vi "Raw_data.vi"(6 "y axis":dbl[](array[numeric]), 9 "dt/df":dbl, 10 "operation (0:open)":T1(ring), 11 "Data path":path) -> (2 "x axis":dbl[](array[numeric]), 3 "y data":dbl[](array[numeric]))   [LabVIEW 2021]
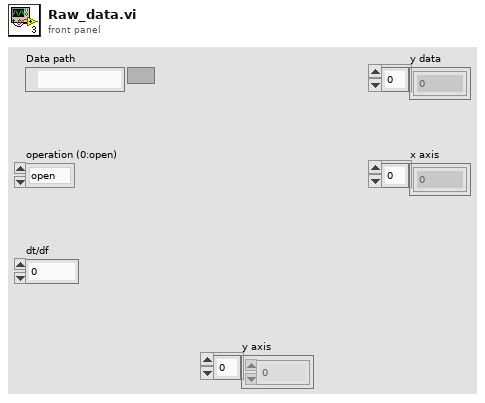
[diagram p1: front panel]
types:
  T1 = enum16{"open", "replace", "create", "open or create", "replace or create", "replace or create with confirmation"}
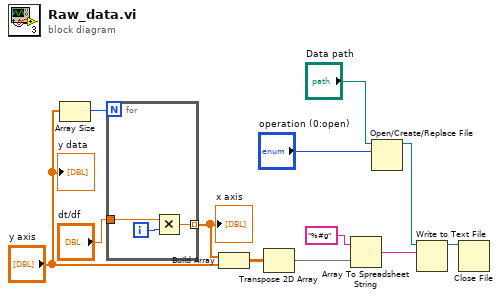
[diagram p0: block diagram]
diagram:
  n1 = Array Size(array="y axis") -> (size(s)=w7:i32)
  n2 = for {
    N: w7 -> [_]
    tunnel: [w15] -> w2 mode=indexing
    tunnel: "dt/df" -> [w13]
    i -> [w14]
    n3 = Multiply(x=w13, y=w14) -> (x*y=w15:dbl)
  }
  "x axis" <- w2
  n4 = Build Array(w2, "y axis") -> (w6:dbl[][])
  n5 = Transpose 2D Array(2D array=w6) -> (transposed array=w5:dbl[][])
  n6 = Array To Spreadsheet String(array=w5, 3:"%#g" ("format string")) -> (spreadsheet string=w8:string)  [unwired: 1 in]
  n7 = Open/Create/Replace File(file path (use dialog)="Data path", operation (0:open)="operation (0:open)") -> (refnum out=w11:refnum<file>)  [unwired: 4 in, 2 out]
  n8 = Write to Text File(file (use dialog)=w11, text=w8) -> (refnum out=w10:refnum<file>)  [unwired: 2 in, 2 out]
  n9 = Close File(refnum=w10) -> ()  [unwired: 1 in, 2 out]
  "y data" <- "y axis"
